vi "Intake Activation.vi"(1 "Lower Limit Switch":bool, 2 "Upper Limit Switch":bool, 3 "Down Button Value":bool, 4 "Up Button Value":bool) -> (0 "Intake Motor Set":dbl)   [LabVIEW 2013]
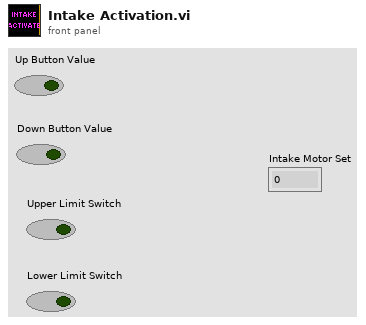
[diagram p1: front panel]
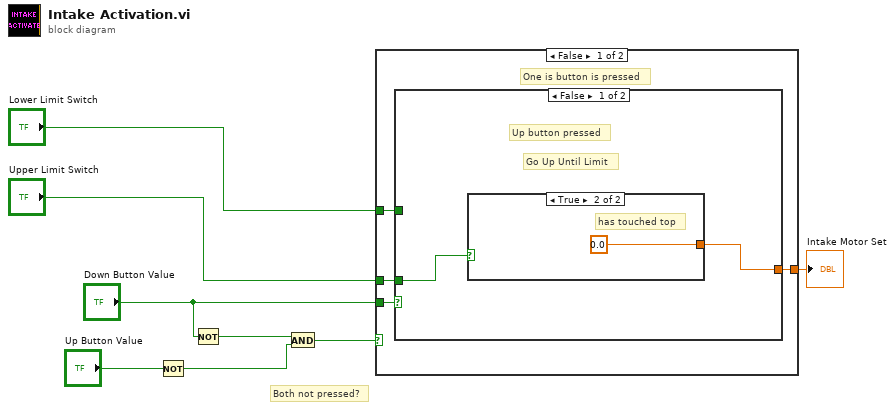
[diagram p0: block diagram]
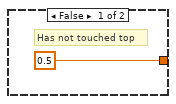
[diagram p2: hidden frame]
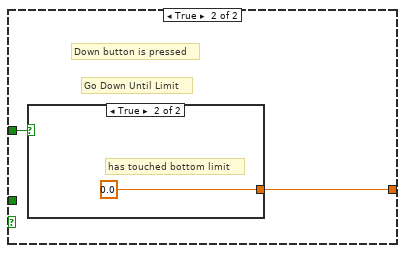
[diagram p3: hidden frame]
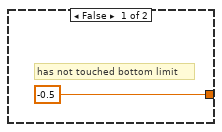
[diagram p4: hidden frame]
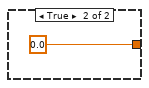
[diagram p5: hidden frame]
diagram:
  # "Both not pressed?"
  n1 = Not(x="Up Button Value") -> (.not. x?=w6:bool)
  n2 = Not(x="Down Button Value") -> (.not. x?=w7:bool)
  n3 = And(x=w7, y=w6) -> (x .and. y?=w8:bool)
  n4 = case shown="False" w8 {
    tunnel: [w9 0.0 ("Output")] -> w1
    tunnel: "Down Button Value" -> [w12 _]
    tunnel: "Upper Limit Switch" -> [w10 _]
    tunnel: "Lower Limit Switch" -> [w11 _]
    frame False {
      # "One is button is pressed"
      n5 = case shown="False" w12 {
        tunnel: w11 -> [_ w18]
        tunnel: w10 -> [w13 _]
        tunnel: [w14 w17] -> w9
        frame False {
          # "Go Up Until Limit"
          # "Up button pressed"
          n6 = case shown="True" w13 {
            tunnel: [0.5 ("Output") 0.0 ("Output")] -> w14
            frame False {
              # "Has not touched top"
            }
            frame True {
              # "has touched top"
            }
          }
        }
        frame True {
          # "Go Down Until Limit"
          # "Down button is pressed"
          n7 = case shown="True" w18 {
            tunnel: [-0.5 ("Output") 0.0 ("Output")] -> w17
            frame False {
              # "has not touched bottom limit"
            }
            frame True {
              # "has touched bottom limit"
            }
          }
        }
      }
    }
    frame True {
    }
  }
  "Intake Motor Set" <- w1
